vi "Untitled 1.vi"() -> ()   [LabVIEW 2020]
panel:
  in  "Numeric 6":dbl
  in  "stop 2":bool
  in  "Numeric 8":dbl
  out "Numeric 7":dbl
  in  "Enum":enum16{"mult", "sup", "add"}(ring)
  out "Boolean":bool
  in  "stop":bool
  out "Numeric 5":i32
  out "Numeric 3":dbl
  in  "Numeric 4":dbl
  in  "String 2":string
  out "String":string
  out "Numeric 2":dbl
  in  "Numeric":dbl
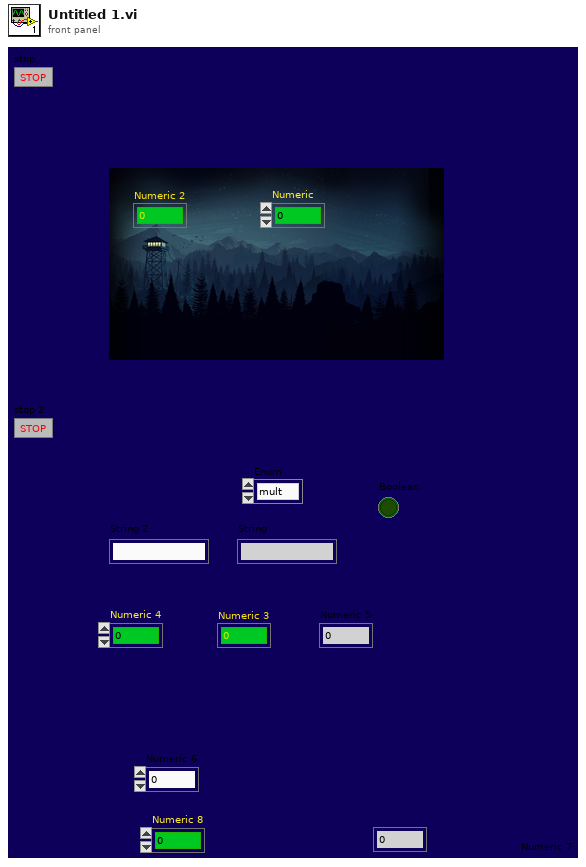
[diagram p1: front panel]
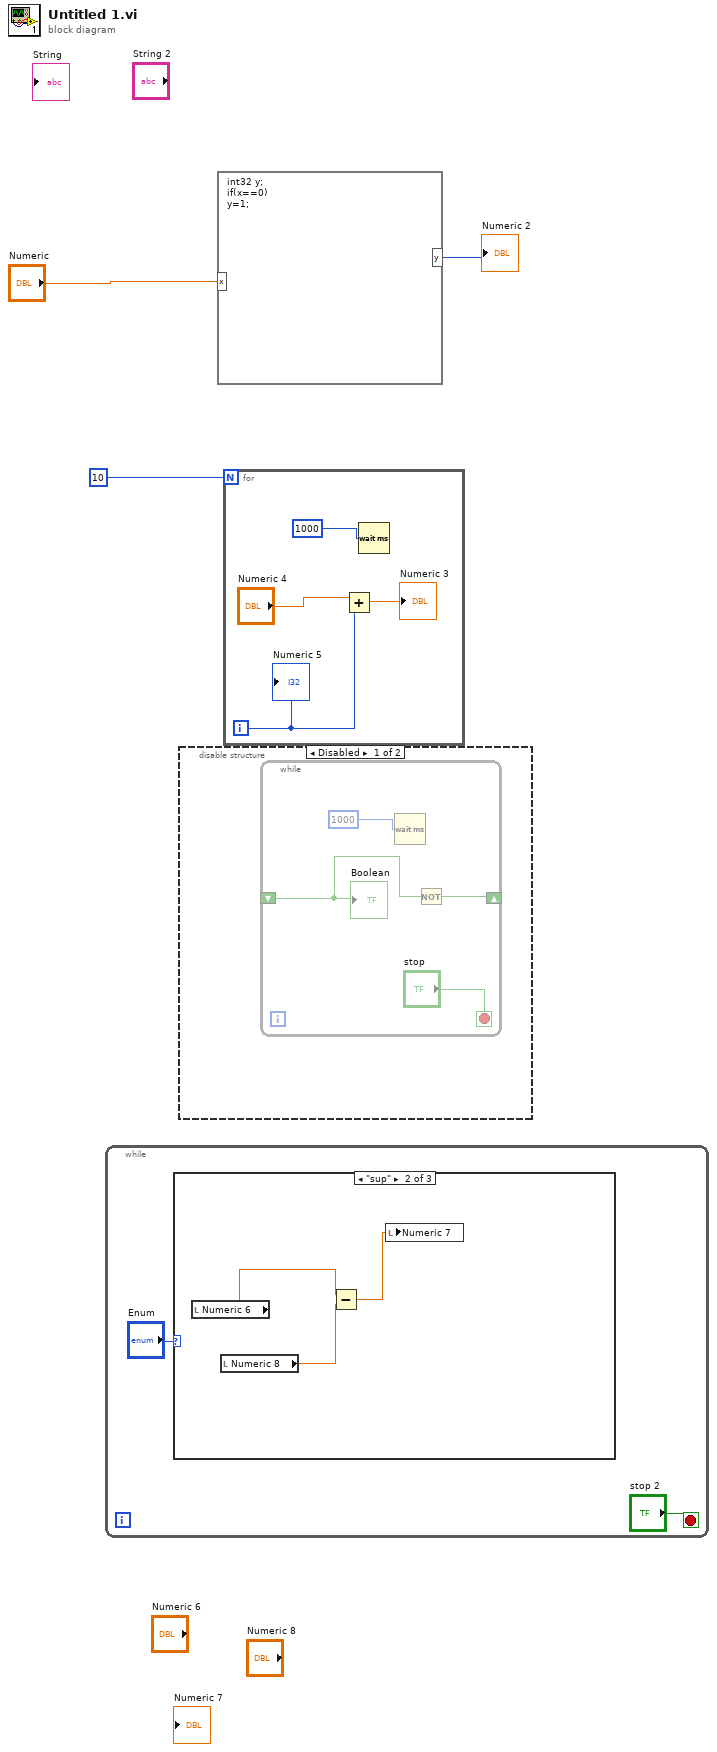
[diagram p0: block diagram]
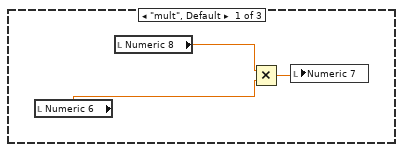
[diagram p2: hidden frame]
diagram:
  n1 = while {
    stop <- "stop 2" stop-if-true
    n2 = case shown="\"sup\"" "Enum" {
      frame "mult", Default {
        n3 = local read "Numeric 6"() -> (w6:dbl)
        n4 = local read "Numeric 8"() -> (w7:dbl)
        n5 = Multiply(x=w7, y=w6) -> (x*y=w8:dbl)
        n6 = local write "Numeric 7"(w8) -> ()
      }
      frame "sup" {
        n7 = local read "Numeric 6"() -> (w10:dbl)
        n8 = local read "Numeric 8"() -> (w11:dbl)
        n9 = Subtract(x=w10, y=w11) -> (x-y=w9:dbl)
        n10 = local write "Numeric 7"(w9) -> ()
      }
      frame "add" {
      }
    }
  }
  n11 = disable-structure shown="Disabled" {
    frame Disabled {
      n12 = while {
        shift-right: [w13] -> _
        shift-left: _ -> [w12]
        stop <- "stop" stop-if-true
        n13 = Wait (ms)(milliseconds to wait=u32 1000 ("millisecond timer value")) -> ()  [unwired: 1 out]
        n14 = Not(x=w12) -> (.not. x?=w13:bool)
        "Boolean" <- w12
      }
    }
    frame Enabled {
    }
  }
  n15 = formula code="int32 y;\nif(x==0)\ny=1;"("x"="Numeric") -> ("y"=→"Numeric 2":i32)
  n16 = for {
    N: 10 -> [_]
    i -> [w18]
    n17 = Add(x="Numeric 4", y=w18) -> (x+y=→"Numeric 3":dbl)
    n18 = Wait (ms)(milliseconds to wait=u32 1000 ("millisecond timer value")) -> ()  [unwired: 1 out]
    "Numeric 5" <- w18
  }
